vi "RfRx计算.vi"(0 "输入数据":dbl[][](array[numeric])=[[199.921, 4.0, 7.8325, 4.0, -2.844e-06, -3.3e-06, -3.109e-06, -3.045e-06, -2.897e-06, 1.0, 0.0], [299.9351, 4.0, 7.8338, 1.0, -3.491e-06, -2.918e-06, -3.332e-06, -2.78e-06, -3.204e-06, 0.0, 0.0], [399.96, 4.0, 7.8346, -3.12e-06, -3.289e-06, -2.96e-06, -3.141e-06, -3.385e-06, -2.844e-06, 0.0, 0.0], [400.0285, -4.0, 7.8346, 0.0, -3.342e-06, -3.162e-06, -3.194e-06, -3.056e-06, -3.194e-06, 0.0, 0.0], [300.0653, -4.0, 7.8332, -3.342e-06, -3.321e-06, -3.013e-06, -3.311e-06, -3.3e-06, -3.162e-06, 0.0, 0.0], [200.0595, -4.0, 7.8346, -2.907e-06, -3.194e-06, -3.257e-06, -3.204e-06, -3.077e-06, -2.971e-06, 0.0, 0.0], [199.9466, 4.0, 8.8568, 5.0, -3.353e-06, -3.799e-06, -3.565e-06, -3.746e-06, -3.374e-06, 0.0, 0.0], [299.95, 4.0, 8.8574, -3.311e-06, -3.502e-06, -3.364e-06, -3.618e-06, -3.12e-06, -3.406e-06, 0.0, 0.0], [399.8962, 4.0, 8.8567, -3.756e-06, -3.83e-06, -3.427e-06, -3.597e-06, -3.777e-06, -3.576e-06, 0.0, 0.0], [399.9835, -4.0, 8.8567, 0.0, -3.289e-06, -3.12e-06, -3.502e-06, -3.427e-06, -3.353e-06, 0.0, 0.0], [299.9459, -4.0, 8.8552, -3.512e-06, -3.65e-06, -3.809e-06, -3.48e-06, -3.3e-06, -3.767e-06, 0.0, 0.0], [199.9841, -4.0, 8.8564, -3.629e-06, -3.608e-06, -3.767e-06, -3.639e-06, -3.417e-06, -3.406e-06, 0.0, 0.0], [200.0, 4.0, 0.0, 1.0, 0.0, 0.0, 0.0, 0.0, 0.0, 0.0, 0.0], [300.0, 4.0, 0.0, 2.0, 0.0, 0.0, 0.0, 0.0, 0.0, 0.0, 0.0], [400.0, 4.0, 0.0, 3.0, 0.0, 0.0, 0.0, 0.0, 0.0, 0.0, 0.0], [400.0, -4.0, 0.0, 20.0, 0.0, 0.0, 0.0, 0.0, 0.0, 0.0, 0.0], [300.0, -4.0, 0.0, 5.0, 0.0, 0.0, 0.0, 0.0, 0.0, 0.0, 0.0], [200.0, -4.0, 0.0, 6.0, 0.0, 0.0, 0.0, 0.0, 0.0, 0.0, 0.0], [200.0, 0.0, 0.0, 7.0, 0.0, 0.0, 0.0, 0.0, 0.0, 0.0, 0.0], [300.0, 0.0, 0.0, 8.0, 0.0, 0.0, 0.0, 0.0, 0.0, 0.0, 0.0], [400.0, 0.0, 0.0, 9.0, 0.0, 0.0, 0.0, 0.0, 0.0, 0.0, 0.0], [400.0, -7.0, 0.0, 10.0, 0.0, 0.0, 0.0, 0.0, 0.0, 0.0, 0.0], [300.0, -7.0, 0.0, 11.0, 0.0, 0.0, 0.0, 0.0, 0.0, 0.0, 0.0], [200.0, -7.0, 0.0, 12.0, 0.0, 0.0, 0.0, 0.0, 0.0, 0.0, 0.0], [0.0, 0.0, 0.0, 13.0, 0.0, 0.0, 0.0, 0.0, 0.0, 0.0, 0.0], [0.0, 0.0, 0.0, 14.0, 0.0, 0.0, 0.0, 0.0, 0.0, 0.0, 0.0], [0.0, 0.0, 0.0, 15.0, 0.0, 0.0, 0.0, 0.0, 0.0, 0.0, 0.0], [0.0, -7.0, 0.0, 16.0, 0.0, 0.0, 0.0, 0.0, 0.0, 0.0, 0.0], [0.0, -7.0, 0.0, 17.0, 0.0, 0.0, 0.0, 0.0, 0.0, 0.0, 0.0], [0.0, -7.0, 0.0, 18.0, 0.0, 0.0, 0.0, 0.0, 0.0, 0.0, 0.0], [0.0, 0.0, 0.0, 19.0, 0.0, 0.0, 0.0, 0.0, 0.0, 0.0, 0.0], [0.0, 0.0, 0.0, 20.0, 0.0, 0.0, 0.0, 0.0, 0.0, 0.0, 0.0], [0.0, 0.0, 0.0, 21.0, 0.0, 0.0, 0.0, 0.0, 0.0, 0.0, 0.0], [0.0, -7.0, 0.0, 22.0, 0.0, 0.0, 0.0, 0.0, 0.0, 0.0, 0.0], [0.0, -7.0, 0.0, 23.0, 0.0, 0.0, 0.0, 0.0, 0.0, 0.0, 0.0], [0.0, -7.0, 0.0, 24.0, 0.0, 0.0, 0.0, 0.0, 0.0, 0.0, 0.0], [0.0, 0.0, 0.0, 25.0, 0.0, 0.0, 0.0, 0.0, 0.0, 0.0, 0.0], [0.0, 0.0, 0.0, 26.0, 0.0, 0.0, 0.0, 0.0, 0.0, 0.0, 0.0], [0.0, 0.0, 0.0, 27.0, 0.0, 0.0, 0.0, 0.0, 0.0, 0.0, 0.0]], 1 "R3-1":dbl[](array[numeric]), 3 "R5-1":dbl[](array[numeric]), 5 "压力点个数":i32=6, 9 "理论K":dbl=306.667, 11 "检定次数":i32=3, 12 "Vx":dbl[](array[numeric]), 13 "RG":dbl[](array[numeric]), 14 "R3-2":dbl[](array[numeric])) -> (4 "Rf":dbl[](array[numeric]), 6 "Rx":dbl[](array[numeric]))   [LabVIEW 2017]
uses:
  6cb689a5-d127-45df-bd26-ec4adf835a4e.vi
  <vilib>/Array/Sort 2D Array - Pop Stack.vi
  <vilib>/Array/Sort 2D Array - Push Stack.vi
  <vilib>/Analysis/NI_AALPro.lvlib
panel:
  in  "数据":dbl[][](array[numeric])=[[199.921, 4.0, 7.8325, 4.0, -2.844e-06, -3.3e-06, -3.109e-06, -3.045e-06, -2.897e-06, 1.0, 0.0], [299.9351, 4.0, 7.8338, 1.0, -3.491e-06, -2.918e-06, -3.332e-06, -2.78e-06, -3.204e-06, 0.0, 0.0], [399.96, 4.0, 7.8346, -3.12e-06, -3.289e-06, -2.96e-06, -3.141e-06, -3.385e-06, -2.844e-06, 0.0, 0.0], [400.0285, -4.0, 7.8346, 0.0, -3.342e-06, -3.162e-06, -3.194e-06, -3.056e-06, -3.194e-06, 0.0, 0.0], [300.0653, -4.0, 7.8332, -3.342e-06, -3.321e-06, -3.013e-06, -3.311e-06, -3.3e-06, -3.162e-06, 0.0, 0.0], [200.0595, -4.0, 7.8346, -2.907e-06, -3.194e-06, -3.257e-06, -3.204e-06, -3.077e-06, -2.971e-06, 0.0, 0.0], [199.9466, 4.0, 8.8568, 5.0, -3.353e-06, -3.799e-06, -3.565e-06, -3.746e-06, -3.374e-06, 0.0, 0.0], [299.95, 4.0, 8.8574, -3.311e-06, -3.502e-06, -3.364e-06, -3.618e-06, -3.12e-06, -3.406e-06, 0.0, 0.0], [399.8962, 4.0, 8.8567, -3.756e-06, -3.83e-06, -3.427e-06, -3.597e-06, -3.777e-06, -3.576e-06, 0.0, 0.0], [399.9835, -4.0, 8.8567, 0.0, -3.289e-06, -3.12e-06, -3.502e-06, -3.427e-06, -3.353e-06, 0.0, 0.0], [299.9459, -4.0, 8.8552, -3.512e-06, -3.65e-06, -3.809e-06, -3.48e-06, -3.3e-06, -3.767e-06, 0.0, 0.0], [199.9841, -4.0, 8.8564, -3.629e-06, -3.608e-06, -3.767e-06, -3.639e-06, -3.417e-06, -3.406e-06, 0.0, 0.0], [200.0, 4.0, 0.0, 1.0, 0.0, 0.0, 0.0, 0.0, 0.0, 0.0, 0.0], [300.0, 4.0, 0.0, 2.0, 0.0, 0.0, 0.0, 0.0, 0.0, 0.0, 0.0], [400.0, 4.0, 0.0, 3.0, 0.0, 0.0, 0.0, 0.0, 0.0, 0.0, 0.0], [400.0, -4.0, 0.0, 20.0, 0.0, 0.0, 0.0, 0.0, 0.0, 0.0, 0.0], [300.0, -4.0, 0.0, 5.0, 0.0, 0.0, 0.0, 0.0, 0.0, 0.0, 0.0], [200.0, -4.0, 0.0, 6.0, 0.0, 0.0, 0.0, 0.0, 0.0, 0.0, 0.0], [200.0, 0.0, 0.0, 7.0, 0.0, 0.0, 0.0, 0.0, 0.0, 0.0, 0.0], [300.0, 0.0, 0.0, 8.0, 0.0, 0.0, 0.0, 0.0, 0.0, 0.0, 0.0], [400.0, 0.0, 0.0, 9.0, 0.0, 0.0, 0.0, 0.0, 0.0, 0.0, 0.0], [400.0, -7.0, 0.0, 10.0, 0.0, 0.0, 0.0, 0.0, 0.0, 0.0, 0.0], [300.0, -7.0, 0.0, 11.0, 0.0, 0.0, 0.0, 0.0, 0.0, 0.0, 0.0], [200.0, -7.0, 0.0, 12.0, 0.0, 0.0, 0.0, 0.0, 0.0, 0.0, 0.0], [0.0, 0.0, 0.0, 13.0, 0.0, 0.0, 0.0, 0.0, 0.0, 0.0, 0.0], [0.0, 0.0, 0.0, 14.0, 0.0, 0.0, 0.0, 0.0, 0.0, 0.0, 0.0], [0.0, 0.0, 0.0, 15.0, 0.0, 0.0, 0.0, 0.0, 0.0, 0.0, 0.0], [0.0, -7.0, 0.0, 16.0, 0.0, 0.0, 0.0, 0.0, 0.0, 0.0, 0.0], [0.0, -7.0, 0.0, 17.0, 0.0, 0.0, 0.0, 0.0, 0.0, 0.0, 0.0], [0.0, -7.0, 0.0, 18.0, 0.0, 0.0, 0.0, 0.0, 0.0, 0.0, 0.0], [0.0, 0.0, 0.0, 19.0, 0.0, 0.0, 0.0, 0.0, 0.0, 0.0, 0.0], [0.0, 0.0, 0.0, 20.0, 0.0, 0.0, 0.0, 0.0, 0.0, 0.0, 0.0], [0.0, 0.0, 0.0, 21.0, 0.0, 0.0, 0.0, 0.0, 0.0, 0.0, 0.0], [0.0, -7.0, 0.0, 22.0, 0.0, 0.0, 0.0, 0.0, 0.0, 0.0, 0.0], [0.0, -7.0, 0.0, 23.0, 0.0, 0.0, 0.0, 0.0, 0.0, 0.0, 0.0], [0.0, -7.0, 0.0, 24.0, 0.0, 0.0, 0.0, 0.0, 0.0, 0.0, 0.0], [0.0, 0.0, 0.0, 25.0, 0.0, 0.0, 0.0, 0.0, 0.0, 0.0, 0.0], [0.0, 0.0, 0.0, 26.0, 0.0, 0.0, 0.0, 0.0, 0.0, 0.0, 0.0], [0.0, 0.0, 0.0, 27.0, 0.0, 0.0, 0.0, 0.0, 0.0, 0.0, 0.0]]
  out "平均":dbl[][](array[numeric])
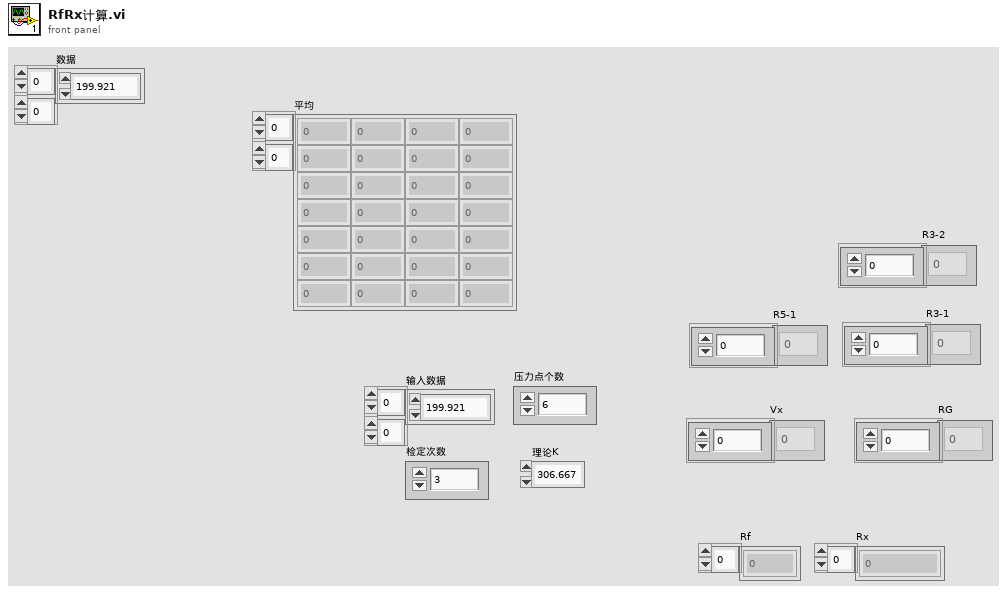
[diagram p1: front panel]
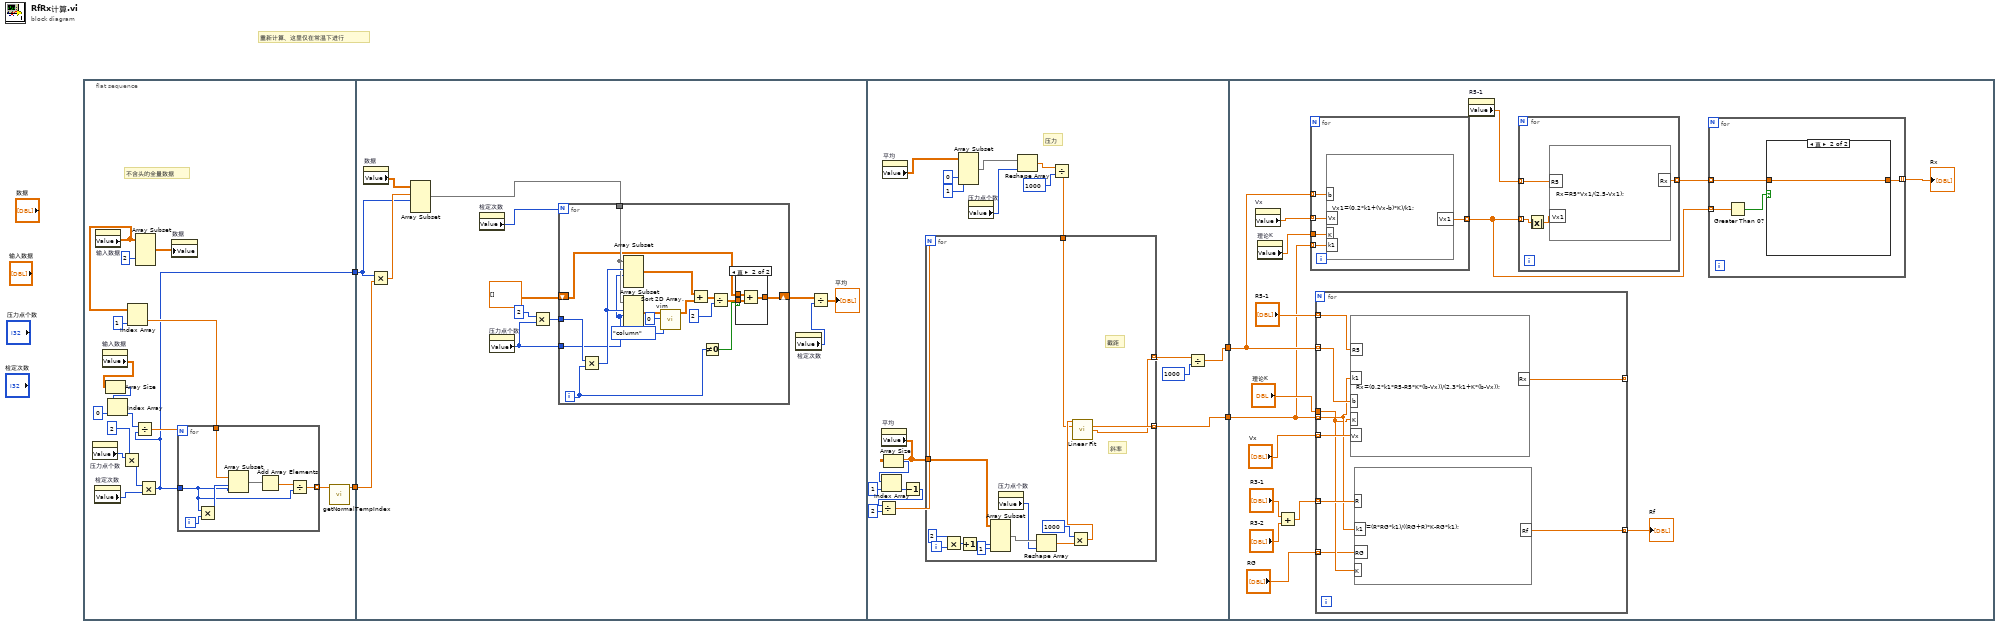
[diagram p0: block diagram]
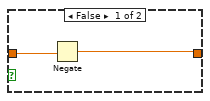
[diagram p3: hidden frame]
diagram:
  # "重新计算、这里仅在常温下进行"
  n1 = flat-sequence {
    tunnel: [w6] -> w2
    tunnel: [w5] -> w1
    tunnel: w2 -> [w32]
    tunnel: w1 -> [w34]
    tunnel: [w63] -> w4
    tunnel: [w65] -> w3
    tunnel: w4 -> [w101]
    tunnel: w3 -> [w100]
    frame #0 {
      # "不含头的全量数据"
      n2 = property on="压力点个数" class="DigNum (严格)"() -> ("Value"=w17:i32)  [unwired: 2 in, 2 out]
      n3 = property on="检定次数" class="DigNum (严格)"() -> ("Value"=w15:i32)  [unwired: 2 in, 2 out]
      n4 = property on="输入数据" class="Arr (严格)"() -> ("Value"=w19:dbl[][])  [unwired: 2 in, 2 out]
      n5 = property on="输入数据" class="Arr (严格)"() -> ("Value"=w12:dbl[][])  [unwired: 2 in, 2 out]
      n6 = Array Size(array=w12) -> (size(s)=w11:i32[])
      n7 = Index Array(array=w11, index=0 ("索引")) -> (element=w10:i32)
      n8 = Multiply(x=w17, y=2) -> (x*y=w14:i32)
      n9 = Index Array(array=w19, index (col)=1 ("禁用的索引 (列)")) -> (element=w8:dbl[])  [unwired: 1 in]
      n10 = Array Subset(array=w19, index (col)=2 ("索引")) -> (w21:dbl[][])  [unwired: 3 in]
      n11 = Multiply(x=w14, y=w15) -> (x*y=w6:i32)
      n12 = Divide(x=w10, y=w6) -> (x/y=w9:dbl)
      n13 = property on="数据" class="Arr (严格)"("Value"=w21) -> ()  [unwired: 2 in, 2 out]
      n14 = for {
        N: w9 -> [_]
        tunnel: w8 -> [w28]
        tunnel: w6 -> [w23]
        tunnel: [w22] -> w7 mode=indexing
        i -> [w27]
        n15 = Multiply(x=w23, y=w27) -> (x*y=w26:i32)
        n16 = Array Subset(array=w28, index=w26, length=w23) -> (w25:dbl[])
        n17 = Add Array Elements(numeric array=w25) -> (sum=w24:dbl)
        n18 = Divide(x=w24, y=w23) -> (x/y=w22:dbl)
      }
      n19 = call "getNormalTempIndex.vi"("温度列表"=w7) -> ("常温索引"=w5:dbl)  [unwired: 10 in]
    }
    frame #1 {
      n20 = property on="数据" class="Arr (严格)"() -> ("Value"=w35:dbl[][])  [unwired: 2 in, 2 out]
      n21 = Multiply(x=w32, y=w34) -> (x*y=w33:dbl)
      n22 = Array Subset(array=w35, index (row)=w33, length (row)=w32) -> (w30:dbl[][])  [unwired: 2 in]
      n23 = property on="检定次数" class="DigNum (严格)"() -> ("Value"=w29:i32)  [unwired: 2 in, 2 out]
      n24 = property on="压力点个数" class="DigNum (严格)"() -> ("Value"=w39:i32)  [unwired: 2 in, 2 out]
      n25 = Multiply(x=2, y=w39) -> (x*y=w40:i32)
      n26 = for {
        N: w29 -> [_]
        tunnel: w40 -> [w57]
        tunnel: w30 -> [w55]
        tunnel: w39 -> [w54]
        shift-right: [w45] -> w37
        shift-left: dbl[][] [] -> [w44]
        i -> [w42]
        n27 = Multiply(x=w57, y=w42) -> (x*y=w56:i32)
        n28 = Array Subset(array=w55, index (row)=w56, length (row)=w54) -> (w49:dbl[][])  [unwired: 2 in]
        n29 = Array Subset(array=w55, index (row)=w56, length (row)=w54) -> (w53:dbl[][])  [unwired: 2 in]
        n30 = call "Sort 2D Array.vim"("index"=0, "dimension to index (column)"=enum16{"column", "row"}."column", "2D array"=w53) -> ("sorted 2D array"=w50:dbl[][])  [unwired: 7 in, 1 out]
        n31 = Add(x=w49, y=w50) -> (x+y=w48:dbl[][])
        n32 = Not Equal To 0?(x=w42) -> (x != 0?=w43:bool)
        n33 = Divide(x=w48, y=2) -> (x/y=w46:dbl[][])
        n34 = case shown="真" w43 {
          tunnel: w46 -> [w58 w61]
          tunnel: [w58 w60] -> w45
          tunnel: w44 -> [_ w59]
          frame False {
          }
          frame True {
            n35 = Add(x=w59, y=w61) -> (x+y=w60:dbl[][])
          }
        }
      }
      n36 = property on="检定次数" class="DigNum (严格)"() -> ("Value"=w31:i32)  [unwired: 2 in, 2 out]
      n37 = Divide(x=w37, y=w31) -> (x/y=→"平均":dbl[][])
    }
    frame #2 {
      # "压力"
      n38 = property on="平均" class="Arr (严格)"() -> ("Value"=w70:dbl[][])  [unwired: 2 in, 2 out]
      n39 = property on="平均" class="Arr (严格)"() -> ("Value"=w77:dbl[][])  [unwired: 2 in, 2 out]
      n40 = Array Size(array=w70) -> (size(s)=w76:i32[])
      n41 = Index Array(array=w76, index=1 ("索引")) -> (element=w75:i32)
      n42 = Decrement(x=w75) -> (x-1=w73:i32)
      n43 = Divide(x=w73, y=2) -> (x/y=w71:dbl)
      n44 = Array Subset(array=w77, index (col)=0 ("索引"), length (col)=1 ("长度")) -> (w78:dbl[][])  [unwired: 2 in]
      n45 = property on="压力点个数" class="DigNum (严格)"() -> ("Value"=w66:i32)  [unwired: 2 in, 2 out]
      n46 = Reshape Array(w78, w66) -> (w69:dbl[])
      n47 = Divide(x=w69, y=1000) -> (x/y=w67:dbl[])
      n48 = for {
        N: w71 -> [_]
        tunnel: w70 -> [w89]
        tunnel: w67 -> [w83]
        tunnel: [w82] -> w65 mode=indexing
        tunnel: [w81] -> w64 mode=indexing
        i -> [w94]
        # "截距"
        # "斜率"
        n49 = Multiply(x=2, y=w94) -> (x*y=w92:i32)
        n50 = Increment(x=w92) -> (x+1=w91:i32)
        n51 = Array Subset(array=w89, index (col)=w91, length (col)=1 ("长度")) -> (w88:dbl[][])  [unwired: 2 in]
        n52 = property on="压力点个数" class="DigNum (严格)"() -> ("Value"=w87:i32)  [unwired: 2 in, 2 out]
        n53 = Reshape Array(w88, w87) -> (w86:dbl[])
        n54 = Multiply(x=1000, y=w86) -> (x*y=w84:dbl[])
        n55 = call <vilib>:"Linear Fit.vi"("Y"=w84, "X"=w83) -> ("slope"=w82:dbl, "intercept"=w81:dbl)  [unwired: 9 in, 3 out]
      }
      n56 = Divide(x=w64, y=1000) -> (x/y=w63:dbl[])
    }
    frame #3 {
      n57 = property on="Vx" class="Arr (严格)"() -> ("Value"=w102:dbl[])  [unwired: 2 in, 2 out]
      n58 = property on="理论K" class="DigNum (严格)"() -> ("Value"=w103:dbl)  [unwired: 2 in, 2 out]
      n59 = Add(x="R3-1", y="R3-2") -> (x+y=w104:dbl[])
      n60 = for {
        tunnel: w103 -> [w126]
        tunnel: w102 -> [w125] mode=indexing
        tunnel: w101 -> [w124] mode=indexing
        tunnel: w100 -> [w123] mode=indexing
        tunnel: [w122] -> w97 mode=indexing
        n61 = formula code="Vx1=(0.2*k1+(Vx-b)*K)/k1;"("Vx"=w125, "b"=w124, "K"=w126, "k1"=w123) -> ("Vx1"=w122:dbl)
      }
      n62 = for {
        tunnel: w101 -> [w133] mode=indexing
        tunnel: w100 -> [w130] mode=indexing
        tunnel: "Vx" -> [w135] mode=indexing
        tunnel: "R5-1" -> [w134] mode=indexing
        tunnel: "理论K" -> [w129]
        tunnel: [w132] -> _ mode=indexing
        tunnel: w104 -> [w131] mode=indexing
        tunnel: "RG" -> [w128] mode=indexing
        tunnel: [w127] -> w96 mode=indexing
        n63 = formula code="Rx=(0.2*k1*R5-R5*K*(b-Vx))/(2.3*k1+K*(b-Vx));"("k1"=w130, "R5"=w134, "K"=w129, "b"=w133, "Vx"=w135) -> ("Rx"=w132:dbl)
        n64 = formula code="Rf=(R*RG*k1)/((RG+R)*K-RG*k1);"("k1"=w130, "R"=w131, "K"=w129, "RG"=w128) -> ("Rf"=w127:dbl)
      }
      "Rf" <- w96
      n65 = property on="R5-1" class="Arr (严格)"() -> ("Value"=w99:dbl[])  [unwired: 2 in, 2 out]
      n66 = for {
        tunnel: w99 -> [w121] mode=indexing
        tunnel: w97 -> [w119] mode=indexing
        tunnel: [w120] -> w98 mode=indexing
        n67 = Absolute Value(x=w119) -> (abs(x)=w118:dbl)
        n68 = formula code="Rx=R5*Vx1/(2.5-Vx1);"("R5"=w121, "Vx1"=w118) -> ("Rx"=w120:dbl)
      }
      n69 = for {
        tunnel: w98 -> [w112] mode=indexing
        tunnel: w97 -> [w114] mode=indexing
        tunnel: [w111] -> w95 mode=indexing
        n70 = Greater Than 0?(x=w114) -> (x > 0?=w113:bool)
        n71 = case shown="真" w113 {
          tunnel: w112 -> [w116 w117]
          tunnel: [w115 w117] -> w111
          frame False {
            n72 = Negate(x=w116) -> (-x=w115:dbl)
          }
          frame True {
          }
        }
      }
      "Rx" <- w95
    }
  }
